vi "FTP_CWD.vi"(0 "connection ID":refnum<k5>, 1 "path":string, 2 "error in":errorcluster) -> (3 "connection ID out":refnum<k5>, 4 "reply string":string, 5 "Good Reply?":bool, 6 "error out":errorcluster)   [LabVIEW 2012]
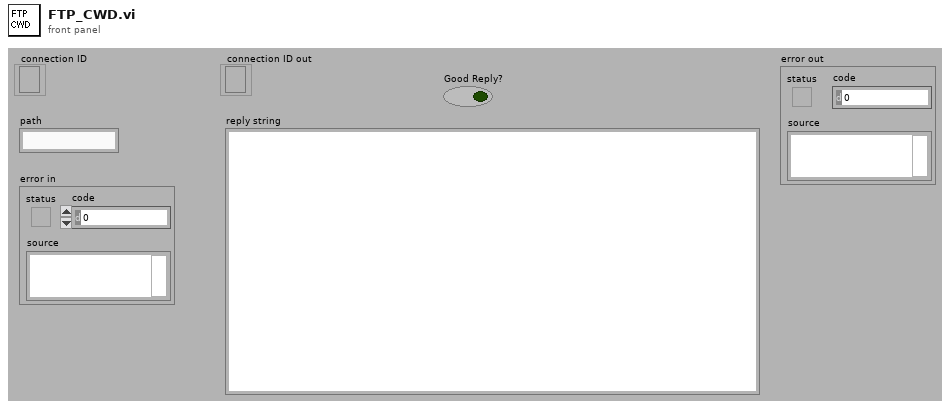
[diagram p1: front panel]
types:
  T1 = enum16{"unknown", "100 + Prelim", "200 + ", "300 + Intermed", "400 - Transient", "500 - Permanent"}
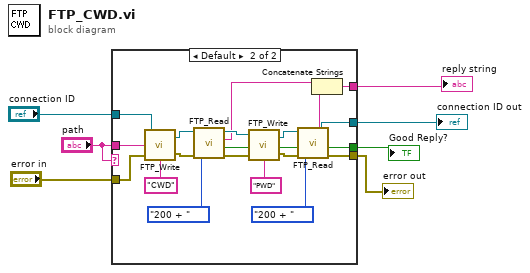
[diagram p0: block diagram]
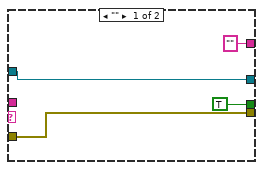
[diagram p2: hidden frame]
diagram:
  n1 = case shown="Default" "path" {
    tunnel: [TRUE ("Good Reply?") w30] -> w7
    tunnel: "path" -> [_ w28]
    tunnel: "error in" -> [w10 w27]
    tunnel: "connection ID" -> [w11 w26]
    tunnel: [w10 w16] -> w4
    tunnel: [w11 w15] -> w3
    tunnel: ["" w12] -> w2
    frame "" {
    }
    frame Default {
      n2 = call <userlib>:"FTP_Write.vi"("Cmd"="CWD", "error in"=w27, "data"=w28, "connection ID in"=w26) -> ("error out"=w24:errorcluster, "connection ID out"=w25:refnum<k5>)
      n3 = call <userlib>:"FTP_Read.vi"("error In"=w24, "expected class"=T1."200 + ", "connection ID"=w25) -> ("error out"=w17:errorcluster, "Good Reply?"=w30:bool, "reply string"=w14:string, "connection ID out"=w18:refnum<k5>)  [unwired: 1 out]
      n4 = call <userlib>:"FTP_Write.vi"("Cmd"="PWD", "error in"=w17, "connection ID in"=w18) -> ("error out"=w21:errorcluster, "connection ID out"=w20:refnum<k5>)  [unwired: 1 in]
      n5 = call <userlib>:"FTP_Read.vi"("error In"=w21, "expected class"=T1."200 + ", "connection ID"=w20) -> ("error out"=w16:errorcluster, "reply string"=w13:string, "connection ID out"=w15:refnum<k5>)  [unwired: 2 out]
      n6 = Concatenate Strings(w14, w13) -> (w12:string)
    }
  }
  "reply string" <- w2
  "Good Reply?" <- w7
  "error out" <- w4
  "connection ID out" <- w3
